vi "Configure IQ vs Slot Measurement Statistics.vi"(7 "Statistic Count (1)":i32=1 format="%.0g", 8 "error in (no error)":errorcluster, 9 "Repetition (Single)":i32(ring) items=["Single", "Continuous"], 10 "Instance (1)":i32=1 format="%.0g", 11 "VISA resource name":refnum<visa-resource-name>) -> (0 "error out":errorcluster, 3 "VISA resource name out":refnum<visa-resource-name>)   [LabVIEW 2015, in "Rohde&Schwarz CMXP GPRF.lvlib"]
doc: "Specifies the scope of the measurement.\n\nAttributes:\nRSCMXPGPRF_ATTR_IQ_VS_SLOT_MEASUREMENT_REPETITION_MODE\nRSCMXPGPRF_ATTR_IQ_VS_SLOT_MEASUREMENT_COUNT\n\nRemote-control commands:\nCONFigure:GPRF:MEAS<i>:IQVSlot:REPetition\nCONFigure:GPRF:MEAS<i>:IQVSlot:SCOunt"
uses:
  <instrlib>/Rohde&Schwarz CMXP GPRF/Rohde&Schwarz CMXP GPRF.lvlib
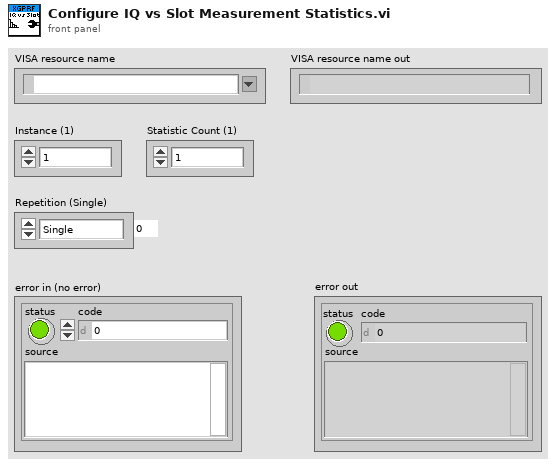
[diagram p1: front panel]
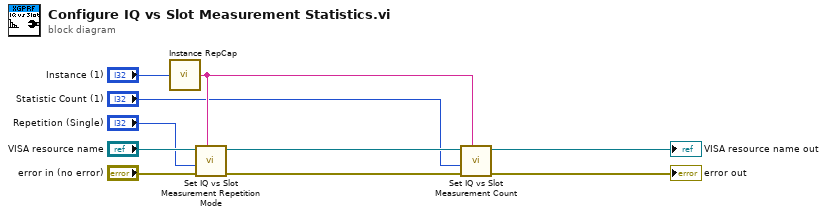
[diagram p0: block diagram]
diagram:
  n1 = call <instrlib>:"Instance RepCap.vi"("instance  in"="Instance (1)") -> ("instance out"=w8:string)
  n2 = call "Set IQ vs Slot Measurement Repetition Mode"("Repeated Capabilities"=w8, "error in (no error)"="error in (no error)", "IQ vs Slot Measurement Repetition Mode (0 - Single)"="Repetition (Single)", "instrument handle"="VISA resource name") -> ("error out"=w9:errorcluster, "instrument handle out"=w10:refnum<visa-resource-name>)  [unwired: 6 in]
  n3 = call "Set IQ vs Slot Measurement Count"("Repeated Capabilities"=w8, "error in (no error)"=w9, "IQ vs Slot Measurement Count (0)"="Statistic Count (1)", "instrument handle"=w10) -> ("error out"=→"error out":errorcluster, "instrument handle out"=→"VISA resource name out":refnum<visa-resource-name>)  [unwired: 6 in]
